vi "File Locations.vi"() -> ()   [LabVIEW 2017]
panel:
  out "lastrun":path=path "C:/Data/Settings/Last Run.txt"
  out "fieldlogfile":path=path "C:/Data/logs/field/fieldlog.txt"
  out "templogfolder":path=path "C:/Data/logs/temperature"
  out "Temporary Files":path=path "C:/Data/temp files"
  out "settingsdir":path=path "C:/Data/Settings"
  out "tempsettings":path=path "C:/Data/Settings/settings.txt"
  out "datadir":path=path "C:/Data"
  out "templogfile":path=path "C:/Data/logs/temperature/templog.txt"
  out "cyrolog":path=path "C:/Data/logs/cryogen/cryogenlog.txt"
  out "appmain":path=path "C:/LabView/Apps/Main v2.00.exe"
  out "main":path=path "C:/LabView/Main/Driver.vi"
  # "LabVIEW directory information"
  # "Data directory information"
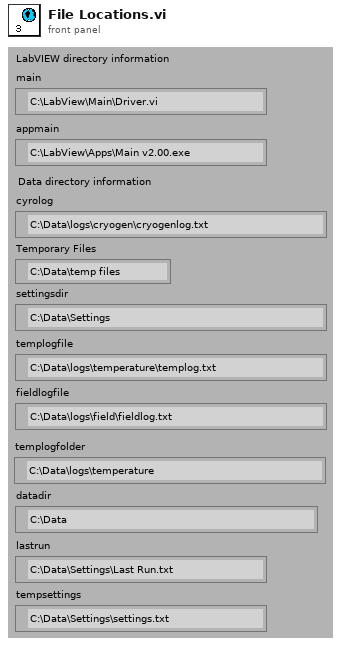
[diagram p1: front panel]
diagram:
